vi "MMC_COM_close.vi"(3 "Error in":errorcluster) -> (0 "Error out":errorcluster, 2 "Close Error Status":bool)   [LabVIEW 2024]
doc: "This Vi terminates serial communication"
uses:
  MMC.dll
panel:
  out "result":i32
  # "MMC_COM_close"
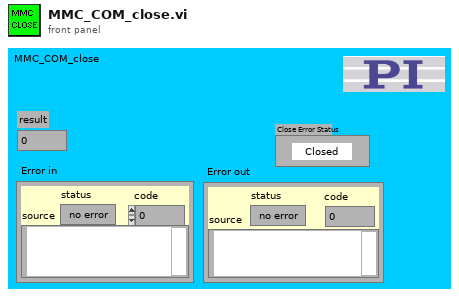
[diagram p1: front panel]
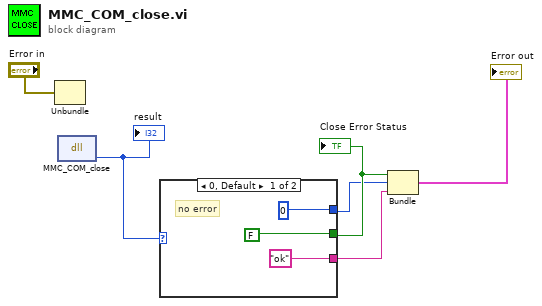
[diagram p0: block diagram]
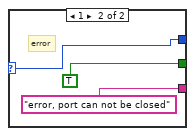
[diagram p2: hidden frame]
diagram:
  n1 = Unbundle("Error in") -> ()  [unwired: 3 out]
  n2 = dll-call lib="E:/Wilson/HoppingSICM_TK/HoppingSICM_v1/DLLs/MMC.dll" fn="MMC_COM_close"() -> ("return type"=w5:u32)  [unwired: 3 in, 2 out]
  "result" <- w5
  n3 = case shown="0, Default" w5 {
    selector: w5 -> [_ w10]
    tunnel: [0 w10] -> w2
    tunnel: [FALSE TRUE] -> w3
    tunnel: ["ok" "error, port can not be closed"] -> w4
    frame 0, Default {
      # "no error"
    }
    frame 1 {
      # "error"
    }
  }
  "Close Error Status" <- w3
  n4 = Bundle(w3, w2, w4) -> (→"Error out":cluster{bool, u32, string})  [unwired: 1 in]
